vi "AdaptToInputs.vi"(3 "Term Types":T1[](array[typedef]), 4 "XRef":refnum<vi>, 5 "State In":T4={"Input Type"=variant(dbl 0.0), "Width"=0, "Typedef Name"="", "Value Type"=variant, "Selection"=0, "Options"=[], "Selections"=[], "Display Selections"=[], "Element Names"=[], "Typedef Name Width"=0, "Display Selection Width"=[], "Code Generated"=FALSE}) -> (0 "Reply":string[](array[string]), 2 "State Out":T4={"Input Type"=variant(dbl 0.0), "Width"=0, "Typedef Name"="", "Value Type"=variant, "Selection"=0, "Options"=[], "Selections"=[], "Display Selections"=[], "Element Names"=[], "Typedef Name Width"=0, "Display Selection Width"=[], "Code Generated"=FALSE})   [LabVIEW 2015, in "Read-Write-Signals.xnode"]
doc: "This ability VI is called by LabVIEW during type propagation so that your XNode may adapt itself to new input types. Term Types is an array of pairs of current Term IDs and the type descriptors corresponding to them. The type descriptors are taken from the signal connected to the terminal. Unwired terminals are not included in the array. Use Reply to inform LabVIEW of any actions it needs to take.\n\nDefault behavior: None.\n\nThis ability does not provide UI and OS messages are not handled."
uses:
  Read-Write-Signals.xnode
  State.ctl
  Read-Write-Signals Item.ctl
  Read-Write-Signals Sub Item.ctl
  Read-Write-Signals Sub Item Type.ctl
  Read-Write-Signals Selection.ctl
  Read-Write-Signals Display Selection.ctl
  <vilib>/XNodeSupport/XNodeTermTypeIDPair.ctl
  <vilib>/XNodeSupport/XNodeType.ctl
  <vilib>/XNodeSupport/XNodeString.ctl
  <vilib>/LV-Scripting/LV-Scripting.lvlib
  <vilib>/Utility/Data Type/NI_Data Type.lvlib
  <vilib>/XNodeSupport/NI_XNodeSupport.lvlib
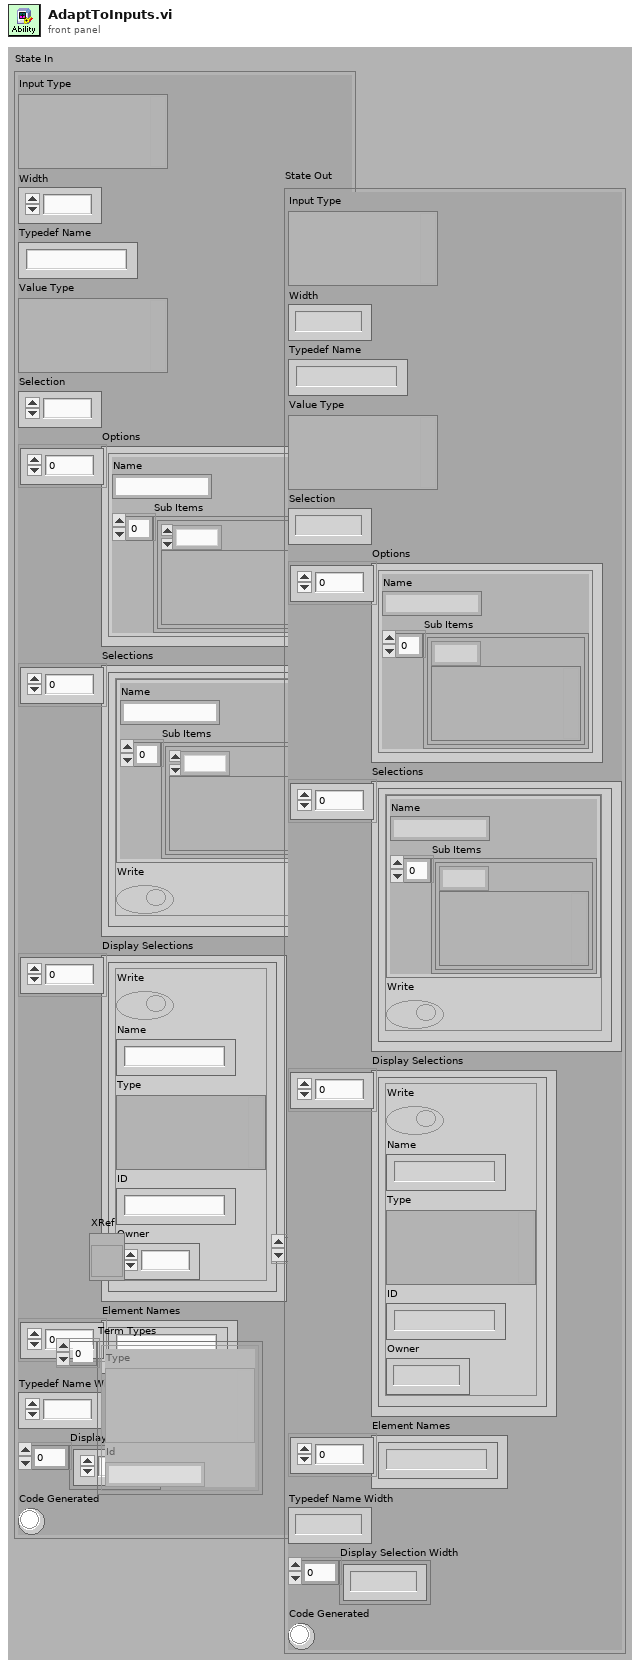
[diagram p1: front panel]
types:
  T1 = typedef "NI_XNodeSupport.lvlib/XNodeTermTypeIDPair.ctl" = cluster{"Type":T2, "Id":T3}
  T2 = typedef "NI_XNodeSupport.lvlib/XNodeType.ctl" = variant
  T3 = typedef "NI_XNodeSupport.lvlib/XNodeString.ctl" = string
  T4 = typedef "Read-Write-Signals.xnode/State.ctl" = cluster{"Input Type":variant, "Width":i32, "Typedef Name":string, "Value Type":variant, "Selection":i32, "Options":T5[], "Selections":T8[], "Display Selections":T9[], "Element Names":string[], "Typedef Name Width":i32, "Display Selection Width":i32[], "Code Generated":bool}
  T5 = typedef "Read-Write-Signals Item.ctl" = cluster{"Name":string, "Sub Items":T6[]}
  T6 = typedef "Read-Write-Signals Sub Item.ctl" = cluster{"Type":T7, "Value":variant}
  T7 = typedef "Read-Write-Signals Sub Item Type.ctl" = enum8{"Cluster Element", "Array Element", "Subarray"}
  T8 = typedef "Read-Write-Signals Selection.ctl" = cluster{"Item":T5, "Write":bool}
  T9 = typedef "Read-Write-Signals Display Selection.ctl" = cluster{"Write":bool, "Name":string, "Type":variant, "ID":string, "Owner":i32}
  T10 = typedef "NI_Data Type.lvlib/Type Definition Info.ctl" = cluster{"Name":string, "Timestamp":u32}
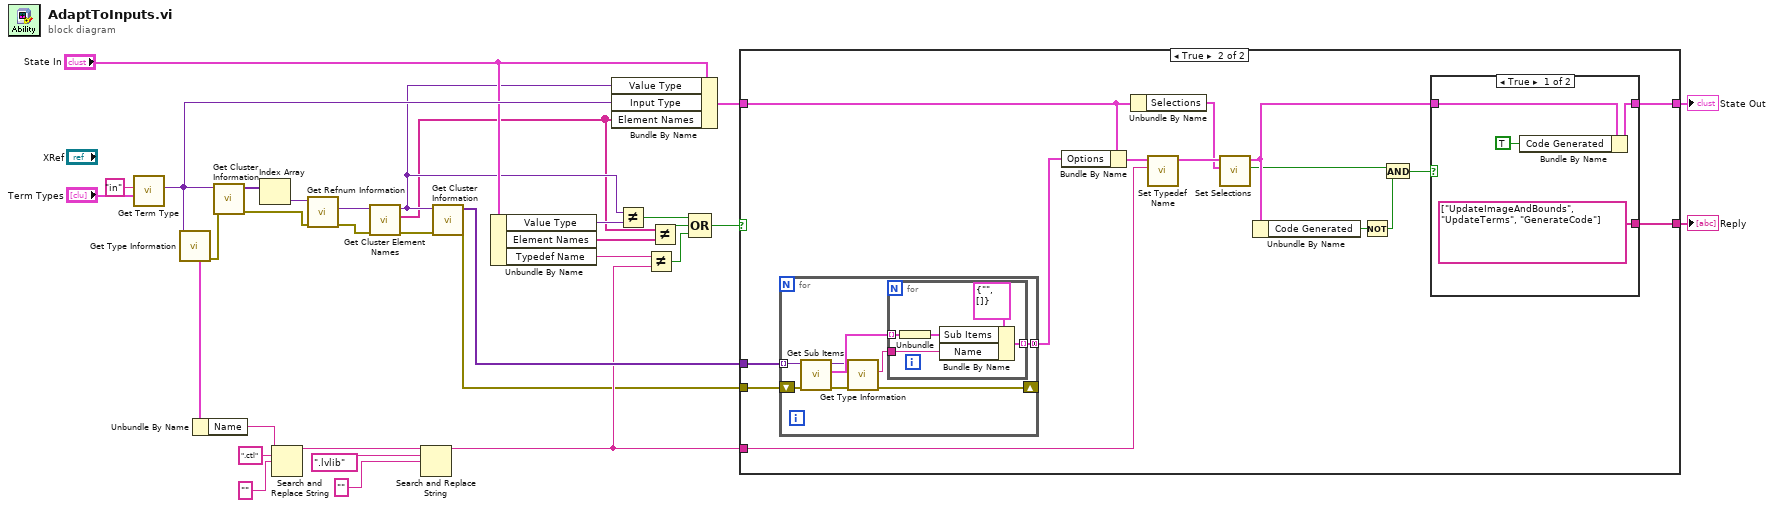
[diagram p0: block diagram]
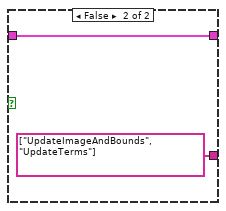
[diagram p3: hidden frame]
diagram:
  n1 = call <vilib>:"Get Term Type.vi"("Term Types"="Term Types", "ID"="in") -> ("Type"=w19:variant)  [unwired: 9 in]
  n2 = call <vilib>:"Get Type Information.vi"("Variant"=w19) -> ("error out"=w27:errorcluster, "Type Definition Info"=w28:T10)  [unwired: 6 in, 3 out]
  n3 = Unbundle By Name(w28) -> ("Name"=w26:string)
  n4 = call <vilib>:"Get Cluster Information.vi"("error in (no error)"=w27, "Variant"=w19) -> ("error out"=w29:errorcluster, "Cluster Elements"=w31:variant[])  [unwired: 8 in]
  n5 = Index Array(array=w31) -> (element=w30:variant)  [unwired: 1 in]
  n6 = Search and Replace String(input string=w26, search string=".ctl", replace string="" ("search string")) -> (result string=w21:string)  [unwired: 5 in, 3 out]
  n7 = call <vilib>:"Get Refnum Information.vi"("error in (no error)"=w29, "Variant"=w30) -> ("error out"=w20:errorcluster, "Strict Type"=w4:variant)  [unwired: 6 in, 2 out]
  n8 = call <vilib>:"Get Cluster Element Names.vi"("error in (no error)"=w20, "Cluster in"=w4) -> ("error out"=w5:errorcluster, "Names"=w2:string[], "Cluster  out"=w3:variant)  [unwired: 7 in]
  n9 = Search and Replace String(input string=w21, search string=".lvlib", replace string="" ("search string")) -> (result string=w6:string)  [unwired: 5 in, 3 out]
  n10 = call <vilib>:"Get Cluster Information.vi"("error in (no error)"=w5, "Variant"=w3) -> ("error out"=w1:errorcluster, "Cluster Elements"=w11:variant[])  [unwired: 8 in]
  n11 = Unbundle By Name("State In") -> ("Value Type"=w17:variant, "Element Names"=w16:string[], "Typedef Name"=w8:string)
  n12 = Bundle By Name(cluster="State In", "Value Type"=w3, "Input Type"=w19, "Element Names"=w2) -> (w10:T4)
  n13 = Not Equal?(x=w3, y=w17) -> (x != y?=w14:bool)
  n14 = Not Equal?(x=w8, y=w6) -> (x != y?=w7:bool)
  n15 = Not Equal?(x=w2, y=w16) -> (x != y?=w15:bool)
  n16 = Compound Arithmetic op=OR(w14, w15, w7) -> (w13:bool)
  n17 = case shown="True" w13 {
    tunnel: [_ w49] -> w12
    tunnel: w11 -> [_ w48]
    tunnel: w10 -> [w34 w42]
    tunnel: [w34 w36] -> w9
    tunnel: w1 -> [_ w46]
    tunnel: w6 -> [_ w43]
    frame False {
    }
    frame True {
      n18 = for {
        tunnel: w48 -> [w61] mode=indexing
        shift-right: [w63] -> _
        shift-left: w46 -> [w59]
        tunnel: [w57] -> w47 mode=concatenating
        n19 = call "Get Sub Items.vi"("error in (no error)"=w59, "Type in"=w61) -> ("error out"=w58:errorcluster, "Sub Items"=w62:cluster{"Sub Items":T6[]}[], "Type out"=w60:variant)  [unwired: 7 in]
        n20 = call <vilib>:"Get Type Information.vi"("error in (no error)"=w58, "Variant"=w60) -> ("error out"=w63:errorcluster, "Name"=w56:string)  [unwired: 5 in, 3 out]
        n21 = for {
          tunnel: w62 -> [w68] mode=indexing
          tunnel: w56 -> [w67]
          tunnel: [w65] -> w57 mode=indexing
          n22 = Unbundle(w68) -> ("Sub Items"=w64:T6[])
          n23 = Bundle By Name(cluster=T5 {"Name"="", "Sub Items"=[]} ("Item"), "Sub Items"=w64, "Name"=w67) -> (w65:T5)
        }
      }
      n24 = Bundle By Name(cluster=w42, "Options"=w47) -> (w44:T4)
      n25 = Unbundle By Name(w42) -> ("Selections"=w41:T8[])
      n26 = call "Set Typedef Name.vi"("Typedef Name"=w43, "State in"=w44) -> ("State out"=w45:T4)  [unwired: 9 in]
      n27 = call "Set Selections.vi"("Selections"=w41, "State in"=w45) -> ("All Valid"=w37:bool, "State out"=w39:T4)  [unwired: 8 in]
      n28 = Unbundle By Name(w39) -> ("Code Generated"=w40:bool)
      n29 = Not(x=w40) -> (.not. x?=w38:bool)
      n30 = And(x=w37, y=w38) -> (x .and. y?=w35:bool)
      n31 = case shown="True" w35 {
        tunnel: [string[] ["UpdateImageAndBounds", "UpdateTerms", "GenerateCode"] ("Reply") string[] ["UpdateImageAndBounds", "UpdateTerms"] ("Reply")] -> w49
        tunnel: w39 -> [w52 w54]
        tunnel: [w51 w54] -> w36
        frame True {
          n32 = Bundle By Name(cluster=w52, "Code Generated"=TRUE) -> (w51:T4)
        }
        frame False {
        }
      }
    }
  }
  "Reply" <- w12
  "State Out" <- w9
